vi "IntroduceSerialNumber.vi"(8 "error in":errorcluster) -> (0 "error out":errorcluster, 3 "Serial Number":string)   [LabVIEW 2009]
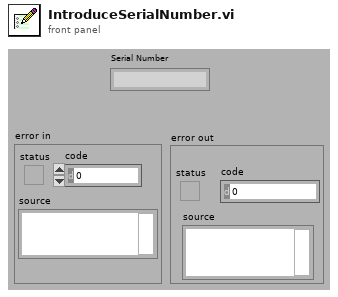
[diagram p1: front panel]
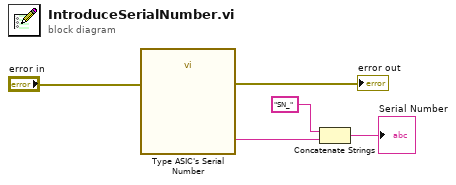
[diagram p0: block diagram]
diagram:
  n1 = call "Type ASIC's Serial Number"("error in (no error)"="error in") -> ("SerialNumber"=w5:string, "error out"=→"error out":errorcluster)  [unwired: 16 in, 1 out]
  n2 = Concatenate Strings("SN_", w5) -> (→"Serial Number":string)
